vi "splitandmerge.vi"() -> ()   [LabVIEW 2017]
uses:
  040-typeDefs/LidarPoint.ctl
  <vilib>/gmath/NI_Gmath.lvlib
panel:
  out "size(s)":i32
  out "Array 2":dbl[](array[numeric])
  out "XY Graph 2":cluster{dbl[], dbl[]}[](graph)
  out "Array":cluster{dbl[], dbl[]}[](array[cluster])
  in  "XYflipped 4":T1[](array[typedef])=[{"X"=-134.98850906315027, "Y"=520.7898831783388}, {"X"=-115.94331762923663, "Y"=526.3821302980621}, {"X"=-97.20615567321154, "Y"=534.228381218403}, {"X"=-76.19267789820181, "Y"=528.5363524249783}, {"X"=-57.53633805116795, "Y"=538.9374451674904}, {"X"=54.6610018064476, "Y"=701.874757261946}, {"X"=82.17232781116256, "Y"=714.2889531149805}, {"X"=112.32780429954543, "Y"=736.4831731826893}, {"X"=805.6667817320254, "Y"=4230.975069273461}, {"X"=1021.7550308782722, "Y"=4464.573513436075}, {"X"=1203.5085597267214, "Y"=4491.555092244168}, {"X"=1405.6718926201302, "Y"=4566.5490833120075}, {"X"=1606.0481210964617, "Y"=4607.086979070671}, {"X"=1288.2556116749497, "Y"=3299.4183546479826}, {"X"=1355.1290527135268, "Y"=3125.9037493966025}, {"X"=1417.516707158832, "Y"=2965.6391191319253}, {"X"=1474.1907079687917, "Y"=2813.1366402182584}, {"X"=1526.593742884797, "Y"=2669.2951399545514}, {"X"=1575.7544663406982, "Y"=2534.0193096753114}, {"X"=1636.6547838240258, "Y"=2427.868431069923}, {"X"=264.50958890512334, "Y"=362.81631354893983}, {"X"=274.59235778929866, "Y"=348.9054843990186}, {"X"=280.1320140475932, "Y"=330.17427929146606}, {"X"=282.6508107508056, "Y"=309.30489679588374}, {"X"=281.22056929813056, "Y"=285.86009061013635}, {"X"=291.5517259914253, "Y"=275.315439217311}, {"X"=296.22488414671705, "Y"=259.78225114942717}, {"X"=290.07404008116634, "Y"=236.07848540472702}, {"X"=297.7685677329387, "Y"=224.63944460017322}, {"X"=301.7354824007149, "Y"=210.6648966021816}, {"X"=300.8805275918088, "Y"=193.99718584576112}, {"X"=304.37784628058256, "Y"=180.74879444575578}, {"X"=302.92213964805364, "Y"=165.11564829247746}, {"X"=304.3190433660061, "Y"=151.62427195142243}, {"X"=303.31765369875154, "Y"=137.43144092486344}, {"X"=317.4249627593629, "Y"=129.96304481358175}, {"X"=316.36091100232704, "Y"=116.12395958534013}, {"X"=317.5683302903703, "Y"=103.47152070297544}, {"X"=326.93101121220707, "Y"=93.36013018287701}, {"X"=319.4646170420994, "Y"=78.63433383799192}, {"X"=326.05907993534385, "Y"=67.63487555778507}, {"X"=328.3275892209375, "Y"=55.58771587650748}, {"X"=751.9447518031435, "Y"=-67.8534467489224}, {"X"=764.8092534665868, "Y"=-97.50797819605364}, {"X"=790.301308999988, "Y"=-130.47927418906556}, {"X"=821.2224333008782, "Y"=-166.84638157114676}, {"X"=839.7964611255854, "Y"=-203.07117934592063}, {"X"=945.348800281241, "Y"=-265.7811991221699}, {"X"=913.0281079276533, "Y"=-293.3609962725949}, {"X"=926.0557331408465, "Y"=-335.62744094750263}, {"X"=2206.2109731110622, "Y"=-892.7671264805506}, {"X"=2149.9546656912585, "Y"=-963.5512106122795}, {"X"=353.36786016387924, "Y"=-174.26174394628646}, {"X"=346.7143217962692, "Y"=-187.15015111229027}]
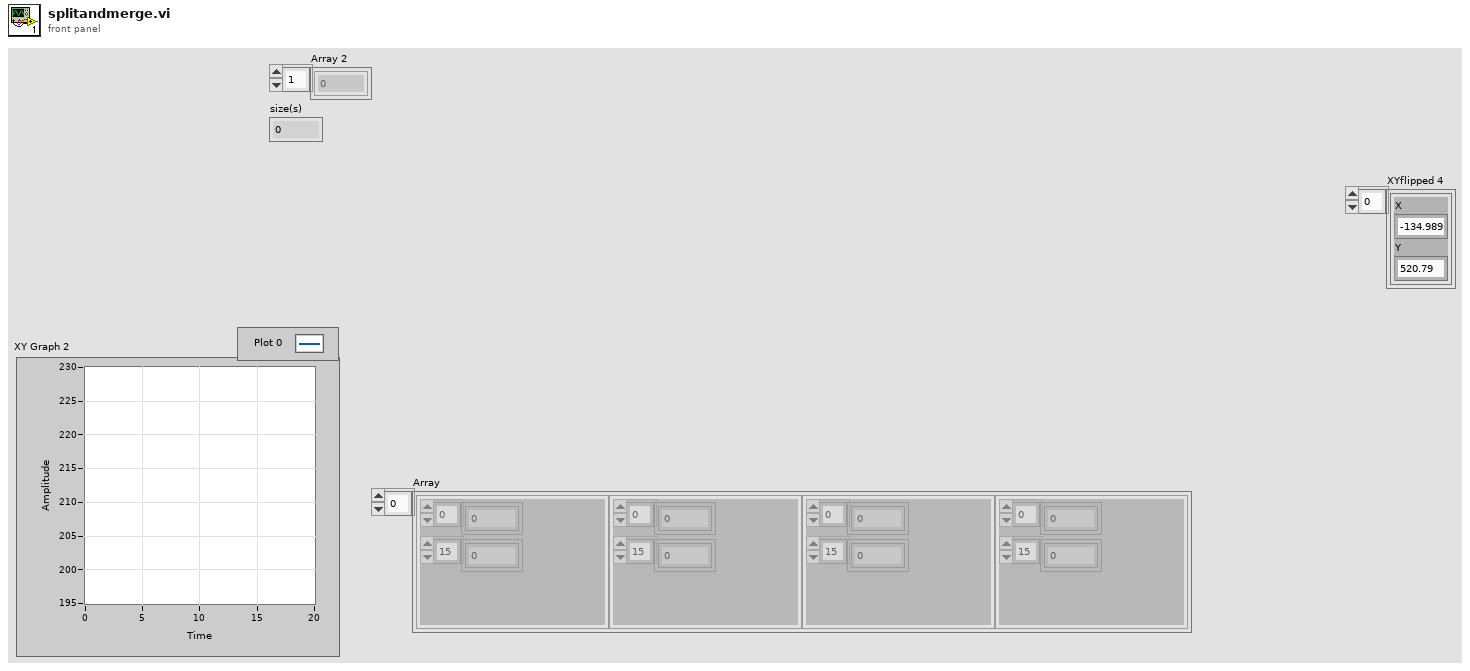
[diagram p1: front panel]
types:
  T1 = typedef "LidarPoint.ctl" = cluster{"X":dbl, "Y":dbl}
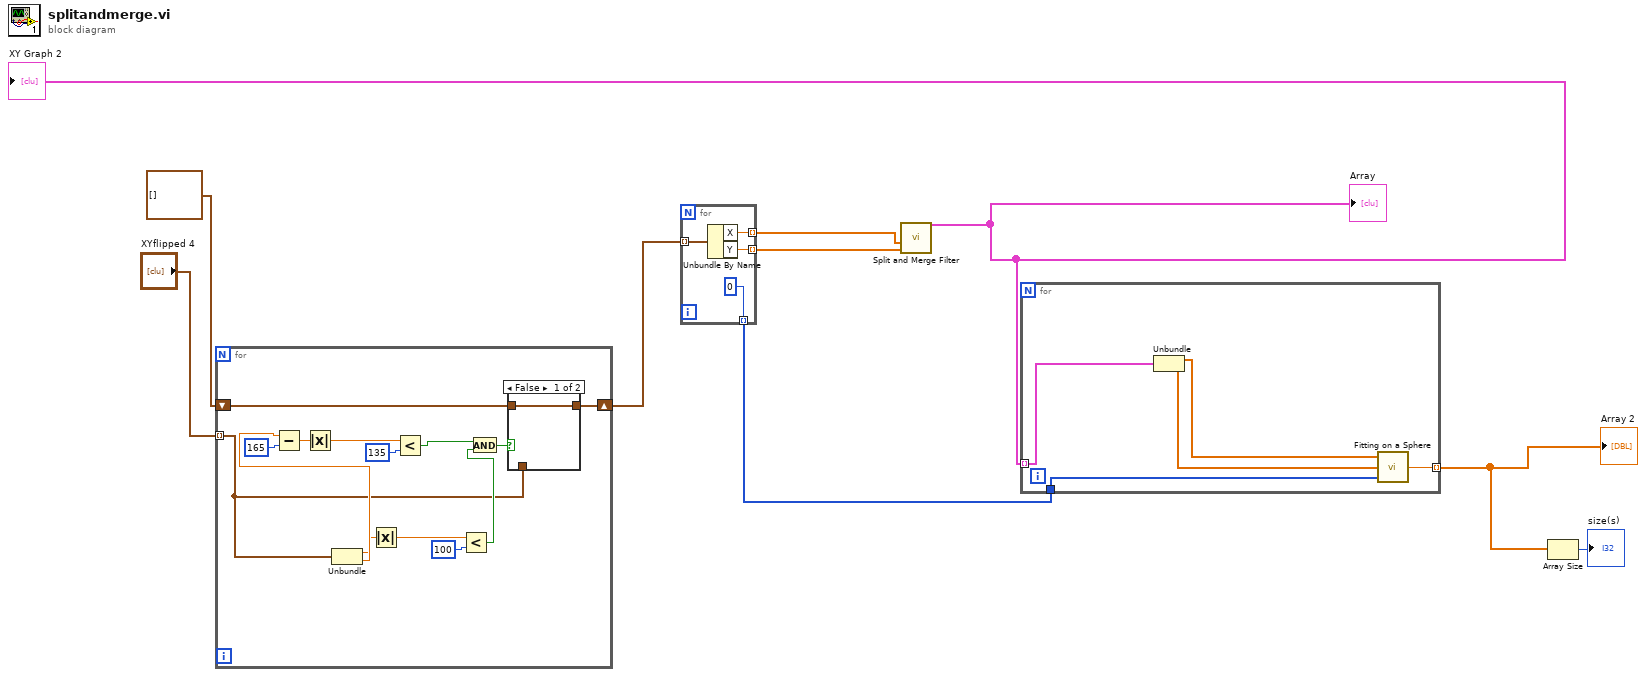
[diagram p0: block diagram]
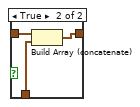
[diagram p2: hidden frame]
diagram:
  n1 = for {
    tunnel: "XYflipped 4" -> [w10] mode=indexing
    shift-right: [w11] -> w7
    shift-left: T1[] [] -> [w20]
    n2 = Unbundle(w10) -> ("X"=w13:dbl, "Y"=w17:dbl)
    n3 = Subtract(x=w17, y=165) -> (x-y=w21:dbl)
    n4 = Absolute Value(x=w21) -> (abs(x)=w22:dbl)
    n5 = Absolute Value(x=w13) -> (abs(x)=w14:dbl)
    n6 = Less?(x=w22, y=135) -> (x < y?=w16:bool)
    n7 = Less?(x=w14, y=100) -> (x < y?=w12:bool)
    n8 = And(x=w16, y=w12) -> (x .and. y?=w19:bool)
    n9 = case shown="False" w19 {
      tunnel: [w24 w27] -> w11
      tunnel: w20 -> [w24 w26]
      tunnel: w10 -> [_ w25]
      frame False {
      }
      frame True {
        n10 = Build Array (concatenate)(w26, w25) -> (w27:T1[])
      }
    }
  }
  n11 = for {
    tunnel: [w31] -> w5 mode=indexing
    tunnel: [w30] -> w6 mode=indexing
    tunnel: w7 -> [w29] mode=indexing
    tunnel: [0] -> w3 mode=indexing
    n12 = Unbundle By Name(w29) -> ("X"=w30:dbl, "Y"=w31:dbl)
  }
  n13 = call "Split and Merge Filter.vi"("Y"=w5, "X"=w6) -> ("Array"=w4:cluster{dbl[], dbl[]}[])  [unwired: 9 in]
  "Array" <- w4
  "XY Graph 2" <- w4
  n14 = for {
    tunnel: w4 -> [w35] mode=indexing
    tunnel: w3 -> [w36]
    tunnel: [w32] -> w2 mode=indexing
    n15 = Unbundle(w35) -> (w34:dbl[], w33:dbl[])
    n16 = call <vilib>:"Fitting on a Sphere.vi"("Z"=w36, "Y"=w33, "X"=w34) -> ("r"=w32:dbl)  [unwired: 2 out]
  }
  "Array 2" <- w2
  n17 = Array Size(array=w2) -> (size(s)=→"size(s)":i32)
